vi "QMH.vi"() -> ()   [LabVIEW 2020]
panel:
  out "Numeric":dbl
  in  "MSG Hnadler":u32
  in  "MSG Producer":u32
  in  "B":dbl format="%#_13g"
  in  "A":dbl format="%#_13g"
  in  "Text Ring":u16(ring) items=["Add", "Sub", "Mul", "Div"]
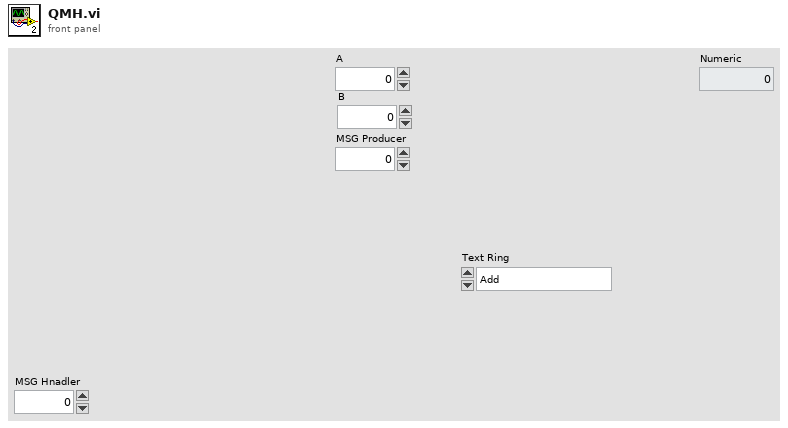
[diagram p1: front panel]
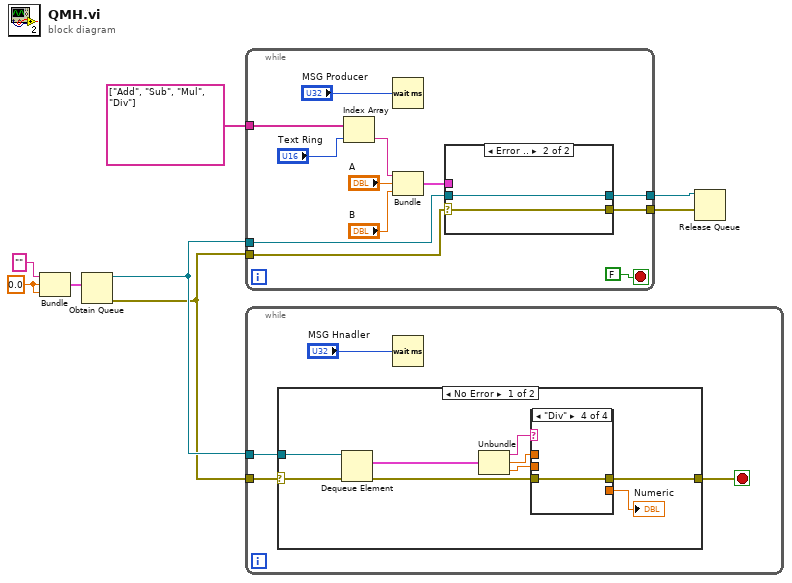
[diagram p0: block diagram]
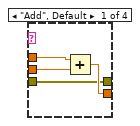
[diagram p2: hidden frame]
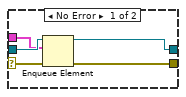
[diagram p6: hidden frame]
diagram:
  w4 = 0.0
  n1 = Bundle("", w4, w4) -> (w3:cluster{string, dbl, dbl})  [unwired: 1 in]
  n2 = Obtain Queue(element data type=w3) -> (queue out=w7:refnum<queue>, error out=w2:errorcluster)  [unwired: 4 in, 1 out]
  n3 = while {
    tunnel: w7 -> [w19]
    tunnel: [w18] -> w8
    tunnel: string[] ["Add", "Sub", "Mul", "Div"] -> [w17]
    tunnel: w2 -> [w10]
    tunnel: [w9] -> w1
    stop <- FALSE stop-if-true
    n4 = Index Array(array=w17, index="Text Ring") -> (element=w14:string)
    n5 = Wait (ms)(milliseconds to wait="MSG Producer") -> ()  [unwired: 1 out]
    n6 = Bundle(w14, "A"="A", "B"="B") -> (w15:cluster{string, "A":dbl, "B":dbl})  [unwired: 1 in]
    n7 = case shown="Error .." w10 {
      selector: w10 -> [w22 w26]
      tunnel: w19 -> [w25 w27]
      tunnel: [w24 w27] -> w18
      tunnel: w15 -> [w23 _]
      tunnel: [w21 w26] -> w9
      frame No Error {
        n8 = Enqueue Element(queue=w25, element=w23, error in (no error)=w22) -> (queue out=w24:refnum<queue>, error out=w21:errorcluster)  [unwired: 1 in, 1 out]
      }
      frame Error {
      }
    }
  }
  n9 = while {
    tunnel: w7 -> [w31]
    tunnel: w2 -> [w29]
    stop <- w28 stop-if-true
    n10 = case shown="No Error" w29 {
      selector: w29 -> [w34 w48]
      tunnel: w31 -> [w40 _]
      tunnel: [w32 w48] -> w28
      frame No Error {
        n11 = Dequeue Element(queue=w40, error in (no error)=w34) -> (element=w39:cluster{string, dbl, dbl}, error out=w33:errorcluster)  [unwired: 1 in, 2 out]
        n12 = Unbundle(w39) -> (w38:string, w37:dbl, w36:dbl)
        n13 = case shown="\"Div\"" w38 {
          tunnel: w37 -> [w44 _ _ _]
          tunnel: w36 -> [w43 _ _ _]
          tunnel: [w42 _ _ _] -> w35
          tunnel: [w41 w45 w46 w47] -> w32
          tunnel: w33 -> [w41 w45 w46 w47]
          frame "Add", Default {
            n14 = Add(x=w44, y=w43) -> (x+y=w42:dbl)
          }
          frame "Sub" {
          }
          frame "Mul" {
          }
          frame "Div" {
          }
        }
        "Numeric" <- w35
      }
      frame Error {
      }
    }
    n15 = Wait (ms)(milliseconds to wait="MSG Hnadler") -> ()  [unwired: 1 out]
  }
  n16 = Release Queue(queue=w8, force destroy? (F)=w1) -> ()  [unwired: 1 in, 3 out]
